vi "myRIO_BRig_RT_dataTrial_SolenoidReward.vi"() -> (2 "output_SolenoidReward":i32)   [LabVIEW 2014]
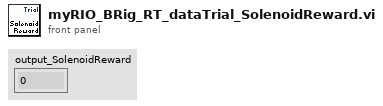
[diagram p1: front panel]
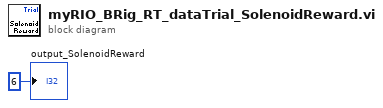
[diagram p0: block diagram]
diagram:
  "output_SolenoidReward" <- 6 ("output_iBlock")
